vi "Global_Device_IDs.vi"() -> ()   [LabVIEW 2017]
uses:
  TypeDef/CLUSTER_Claw_Setup.ctl
  TypeDef/CLUSTER_PWM Motor Setup.ctl
  TypeDef/CLUSTER_Solonoid_Setup.ctl
  <vilib>/Rock Robotics/WPI/Solenoid/WPI_SolenoidChannel.ctl
  <vilib>/Rock Robotics/SystemInterfaces/DIO/FPGA_DIOChannel.ctl
  TypeDef/CLUSTER_Arm_Device_IDs.ctl
  TypeDef/CLUSTER_Talon_Setup.ctl
  _SHARE ALL/RoboRio Share All/SRX Share All/TypeDefs SRX/Cluster_SRX_OPEN Data.ctl
  _SHARE ALL/RoboRio Share All/SRX Share All/TypeDefs SRX/Cluster_SRX_Current Config.ctl
  _SHARE ALL/RoboRio Share All/SRX Share All/TypeDefs SRX/Cluster_SRX_Sensor Config.ctl
  System Drivers/Phoenix-LabVIEW/Motor Controller/Controls/CTRE_Phoenix_MotorControl_FeedbackDevice.ctl
  _SHARE ALL/RoboRio Share All/SRX Share All/TypeDefs SRX/Cluster_SRX_Config Hard Limits.ctl
  System Drivers/Phoenix-LabVIEW/Motor Controller/Controls/CTRE_Phoenix_MotorControl_LimitSwitchNormal.ctl
  _SHARE ALL/RoboRio Share All/SRX Share All/TypeDefs SRX/Cluster_SRX_Motion Magic Config Data.ctl
  _SHARE ALL/RoboRio Share All/SRX Share All/TypeDefs SRX/Cluster_SRX_PIDF.ctl
  _SHARE ALL/RoboRio Share All/SRX Share All/TypeDefs SRX/Cluster_SRX_Config Soft Limits.ctl
  _SHARE ALL/RoboRio Share All/SRX Share All/TypeDefs SRX/Cluster_SRX_Config Voltage Output.ctl
  System Drivers/Phoenix-LabVIEW/Motor Controller/Controls/CTRE_Phoenix_MotorControl_NeutralMode.ctl
  _SHARE ALL/RoboRio Share All/SRX Share All/TypeDefs SRX/Cluster_SRX_Forward and Reverse.ctl
  TypeDef/CLUSTER_Drive_Setup.ctl
panel:
  in  "Drive Setup":T1={"Left Master"={"Open Data"={"SRX ID"=0, "Invert Output"=FALSE}, "Current Config Data"={"Enable Current Limit?"=FALSE, "Peak Current (Amps)"=0, "Peak Current Maximum Duration (ms)"=0, "Continuous Current Limit (Amps)"=0}, "Sensor Config"={"Feedback Device"=1, "PhaseSensor"=FALSE}, "Hard Limits"={"Fwd Enable"=FALSE, "Rev Enable"=FALSE, "Fwd NO-NC"=enum."Normally Open", "Rev NO-NC"=enum."Normally Open"}, "Motion Magic Config Data"={"Cruise Velocity"=0, "Acceleration"=0}, "PIDF"={"P"=0.0, "I"=0.0, "D"=0.0, "F"=0.0, "I Zone"=0.0}, "Maximum Integral Accumulator Value"=0.0, "AllowableClosedLoop"=0, "Limits"={"Max"=0, "Min"=0, "Max Enable"=FALSE, "Min Enable"=FALSE}, "Output Config"={"Invert?"=FALSE, "Neutral Mode"=enum."EEPROMSetting", "Deadband (-1to1)"=0.0, "Ramp Time Off to Full (S)"=0.0, "Peak  (-1to1)"={"Forward"=1.0, "Reverse"=-1.0}, "Nominal  (-1to1)"={"Forward"=0.0, "Reverse"=0.0}}}, "Right Master"={"Open Data"={"SRX ID"=0, "Invert Output"=FALSE}, "Current Config Data"={"Enable Current Limit?"=FALSE, "Peak Current (Amps)"=0, "Peak Current Maximum Duration (ms)"=0, "Continuous Current Limit (Amps)"=0}, "Sensor Config"={"Feedback Device"=1, "PhaseSensor"=FALSE}, "Hard Limits"={"Fwd Enable"=FALSE, "Rev Enable"=FALSE, "Fwd NO-NC"=enum."Normally Open", "Rev NO-NC"=enum."Normally Open"}, "Motion Magic Config Data"={"Cruise Velocity"=0, "Acceleration"=0}, "PIDF"={"P"=0.0, "I"=0.0, "D"=0.0, "F"=0.0, "I Zone"=0.0}, "Maximum Integral Accumulator Value"=0.0, "AllowableClosedLoop"=0, "Limits"={"Max"=0, "Min"=0, "Max Enable"=FALSE, "Min Enable"=FALSE}, "Output Config"={"Invert?"=FALSE, "Neutral Mode"=enum."EEPROMSetting", "Deadband (-1to1)"=0.0, "Ramp Time Off to Full (S)"=0.0, "Peak  (-1to1)"={"Forward"=1.0, "Reverse"=-1.0}, "Nominal  (-1to1)"={"Forward"=0.0, "Reverse"=0.0}}}, "Left Slave"={"Open Data"={"SRX ID"=0, "Invert Output"=FALSE}, "Current Config Data"={"Enable Current Limit?"=FALSE, "Peak Current (Amps)"=0, "Peak Current Maximum Duration (ms)"=0, "Continuous Current Limit (Amps)"=0}, "Sensor Config"={"Feedback Device"=1, "PhaseSensor"=FALSE}, "Hard Limits"={"Fwd Enable"=FALSE, "Rev Enable"=FALSE, "Fwd NO-NC"=enum."Normally Open", "Rev NO-NC"=enum."Normally Open"}, "Motion Magic Config Data"={"Cruise Velocity"=0, "Acceleration"=0}, "PIDF"={"P"=0.0, "I"=0.0, "D"=0.0, "F"=0.0, "I Zone"=0.0}, "Maximum Integral Accumulator Value"=0.0, "AllowableClosedLoop"=0, "Limits"={"Max"=0, "Min"=0, "Max Enable"=FALSE, "Min Enable"=FALSE}, "Output Config"={"Invert?"=FALSE, "Neutral Mode"=enum."EEPROMSetting", "Deadband (-1to1)"=0.0, "Ramp Time Off to Full (S)"=0.0, "Peak  (-1to1)"={"Forward"=1.0, "Reverse"=-1.0}, "Nominal  (-1to1)"={"Forward"=0.0, "Reverse"=0.0}}}, "Right Slave"={"Open Data"={"SRX ID"=0, "Invert Output"=FALSE}, "Current Config Data"={"Enable Current Limit?"=FALSE, "Peak Current (Amps)"=0, "Peak Current Maximum Duration (ms)"=0, "Continuous Current Limit (Amps)"=0}, "Sensor Config"={"Feedback Device"=1, "PhaseSensor"=FALSE}, "Hard Limits"={"Fwd Enable"=FALSE, "Rev Enable"=FALSE, "Fwd NO-NC"=enum."Normally Open", "Rev NO-NC"=enum."Normally Open"}, "Motion Magic Config Data"={"Cruise Velocity"=0, "Acceleration"=0}, "PIDF"={"P"=0.0, "I"=0.0, "D"=0.0, "F"=0.0, "I Zone"=0.0}, "Maximum Integral Accumulator Value"=0.0, "AllowableClosedLoop"=0, "Limits"={"Max"=0, "Min"=0, "Max Enable"=FALSE, "Min Enable"=FALSE}, "Output Config"={"Invert?"=FALSE, "Neutral Mode"=enum."EEPROMSetting", "Deadband (-1to1)"=0.0, "Ramp Time Off to Full (S)"=0.0, "Peak  (-1to1)"={"Forward"=1.0, "Reverse"=-1.0}, "Nominal  (-1to1)"={"Forward"=0.0, "Reverse"=0.0}}}, "Left Slave Top"={"Open Data"={"SRX ID"=0, "Invert Output"=FALSE}, "Current Config Data"={"Enable Current Limit?"=FALSE, "Peak Current (Amps)"=0, "Peak Current Maximum Duration (ms)"=0, "Continuous Current Limit (Amps)"=0}, "Sensor Config"={"Feedback Device"=1, "PhaseSensor"=FALSE}, "Hard Limits"={"Fwd Enable"=FALSE, "Rev Enable"=FALSE, "Fwd NO-NC"=enum."Normally Open", "Rev NO-NC"=enum."Normally Open"}, "Motion Magic Config Data"={"Cruise Velocity"=0, "Acceleration"=0}, "PIDF"={"P"=0.0, "I"=0.0, "D"=0.0, "F"=0.0, "I Zone"=0.0}, "Maximum Integral Accumulator Value"=0.0, "AllowableClosedLoop"=0, "Limits"={"Max"=0, "Min"=0, "Max Enable"=FALSE, "Min Enable"=FALSE}, "Output Config"={"Invert?"=FALSE, "Neutral Mode"=enum."EEPROMSetting", "Deadband (-1to1)"=0.0, "Ramp Time Off to Full (S)"=0.0, "Peak  (-1to1)"={"Forward"=1.0, "Reverse"=-1.0}, "Nominal  (-1to1)"={"Forward"=0.0, "Reverse"=0.0}}}, "Right Slave Top"={"Open Data"={"SRX ID"=0, "Invert Output"=FALSE}, "Current Config Data"={"Enable Current Limit?"=FALSE, "Peak Current (Amps)"=0, "Peak Current Maximum Duration (ms)"=0, "Continuous Current Limit (Amps)"=0}, "Sensor Config"={"Feedback Device"=1, "PhaseSensor"=FALSE}, "Hard Limits"={"Fwd Enable"=FALSE, "Rev Enable"=FALSE, "Fwd NO-NC"=enum."Normally Open", "Rev NO-NC"=enum."Normally Open"}, "Motion Magic Config Data"={"Cruise Velocity"=0, "Acceleration"=0}, "PIDF"={"P"=0.0, "I"=0.0, "D"=0.0, "F"=0.0, "I Zone"=0.0}, "Maximum Integral Accumulator Value"=0.0, "AllowableClosedLoop"=0, "Limits"={"Max"=0, "Min"=0, "Max Enable"=FALSE, "Min Enable"=FALSE}, "Output Config"={"Invert?"=FALSE, "Neutral Mode"=enum."EEPROMSetting", "Deadband (-1to1)"=0.0, "Ramp Time Off to Full (S)"=0.0, "Peak  (-1to1)"={"Forward"=1.0, "Reverse"=-1.0}, "Nominal  (-1to1)"={"Forward"=0.0, "Reverse"=0.0}}}} {"Right Slave Top"."Sensor Config"."Feedback Device" items=["None"=-1, "QuadEncoder"=0, "Analog"=2, "Tachometer"=4, "Pulse Width Encoded Position"=8, "Sensor Sum (S0 + S1)"=9, "Sensor Difference (D0 - D1)"=10, "Remote Source 0"=11, "Remote Source 1"=12, "Software Emulated"=15]; "Left Slave Top"."Sensor Config"."Feedback Device" items=["None"=-1, "QuadEncoder"=0, "Analog"=2, "Tachometer"=4, "Pulse Width Encoded Position"=8, "Sensor Sum (S0 + S1)"=9, "Sensor Difference (D0 - D1)"=10, "Remote Source 0"=11, "Remote Source 1"=12, "Software Emulated"=15]; "Left Master"."Sensor Config"."Feedback Device" items=["None"=-1, "QuadEncoder"=0, "Analog"=2, "Tachometer"=4, "Pulse Width Encoded Position"=8, "Sensor Sum (S0 + S1)"=9, "Sensor Difference (D0 - D1)"=10, "Remote Source 0"=11, "Remote Source 1"=12, "Software Emulated"=15]; "Right Master"."Sensor Config"."Feedback Device" items=["None"=-1, "QuadEncoder"=0, "Analog"=2, "Tachometer"=4, "Pulse Width Encoded Position"=8, "Sensor Sum (S0 + S1)"=9, "Sensor Difference (D0 - D1)"=10, "Remote Source 0"=11, "Remote Source 1"=12, "Software Emulated"=15]; "Left Slave"."Sensor Config"."Feedback Device" items=["None"=-1, "QuadEncoder"=0, "Analog"=2, "Tachometer"=4, "Pulse Width Encoded Position"=8, "Sensor Sum (S0 + S1)"=9, "Sensor Difference (D0 - D1)"=10, "Remote Source 0"=11, "Remote Source 1"=12, "Software Emulated"=15]; "Right Slave"."Sensor Config"."Feedback Device" items=["None"=-1, "QuadEncoder"=0, "Analog"=2, "Tachometer"=4, "Pulse Width Encoded Position"=8, "Sensor Sum (S0 + S1)"=9, "Sensor Difference (D0 - D1)"=10, "Remote Source 0"=11, "Remote Source 1"=12, "Software Emulated"=15]}
  out "Claw Rotation Setup":T2={"Open Data"={"SRX ID"=0, "Invert Output"=FALSE}, "Current Config Data"={"Enable Current Limit?"=FALSE, "Peak Current (Amps)"=0, "Peak Current Maximum Duration (ms)"=0, "Continuous Current Limit (Amps)"=0}, "Sensor Config"={"Feedback Device"=0, "PhaseSensor"=FALSE}, "Hard Limits"={"Fwd Enable"=FALSE, "Rev Enable"=FALSE, "Fwd NO-NC"=enum."Normally Open", "Rev NO-NC"=enum."Normally Open"}, "Motion Magic Config Data"={"Cruise Velocity"=0, "Acceleration"=0}, "PIDF"={"P"=0.0, "I"=0.0, "D"=0.0, "F"=0.0, "I Zone"=0.0}, "Maximum Integral Accumulator Value"=0.0, "AllowableClosedLoop"=0, "Limits"={"Max"=0, "Min"=0, "Max Enable"=FALSE, "Min Enable"=FALSE}, "Output Config"={"Invert?"=FALSE, "Neutral Mode"=enum."Override to Coast", "Deadband (-1to1)"=0.0, "Ramp Time Off to Full (S)"=0.0, "Peak  (-1to1)"={"Forward"=1.0, "Reverse"=-1.0}, "Nominal  (-1to1)"={"Forward"=0.0, "Reverse"=0.0}}} {"Sensor Config"."Feedback Device" items=["None"=-1, "QuadEncoder"=0, "Analog"=2, "Tachometer"=4, "Pulse Width Encoded Position"=8, "Sensor Sum (S0 + S1)"=9, "Sensor Difference (D0 - D1)"=10, "Remote Source 0"=11, "Remote Source 1"=12, "Software Emulated"=15]}
  in  "Lift Setup":T15={"Master"={"Open Data"={"SRX ID"=0, "Invert Output"=FALSE}, "Current Config Data"={"Enable Current Limit?"=FALSE, "Peak Current (Amps)"=0, "Peak Current Maximum Duration (ms)"=2, "Continuous Current Limit (Amps)"=0}, "Sensor Config"={"Feedback Device"=0, "PhaseSensor"=FALSE}, "Hard Limits"={"Fwd Enable"=FALSE, "Rev Enable"=FALSE, "Fwd NO-NC"=enum."Normally Open", "Rev NO-NC"=enum."Normally Open"}, "Motion Magic Config Data"={"Cruise Velocity"=0, "Acceleration"=0}, "PIDF"={"P"=0.0, "I"=0.0, "D"=0.0, "F"=0.0, "I Zone"=0.0}, "Maximum Integral Accumulator Value"=0.0, "AllowableClosedLoop"=0, "Limits"={"Max"=0, "Min"=0, "Max Enable"=FALSE, "Min Enable"=FALSE}, "Output Config"={"Invert?"=FALSE, "Neutral Mode"=enum."Override to Coast", "Deadband (-1to1)"=0.0, "Ramp Time Off to Full (S)"=0.0, "Peak  (-1to1)"={"Forward"=1.0, "Reverse"=-1.0}, "Nominal  (-1to1)"={"Forward"=0.0, "Reverse"=0.0}}}, "Slave"={"Open Data"={"SRX ID"=0, "Invert Output"=FALSE}, "Current Config Data"={"Enable Current Limit?"=FALSE, "Peak Current (Amps)"=0, "Peak Current Maximum Duration (ms)"=-1, "Continuous Current Limit (Amps)"=0}, "Sensor Config"={"Feedback Device"=0, "PhaseSensor"=FALSE}, "Hard Limits"={"Fwd Enable"=FALSE, "Rev Enable"=FALSE, "Fwd NO-NC"=enum."Normally Open", "Rev NO-NC"=enum."Normally Open"}, "Motion Magic Config Data"={"Cruise Velocity"=0, "Acceleration"=0}, "PIDF"={"P"=0.0, "I"=0.0, "D"=0.0, "F"=0.0, "I Zone"=0.0}, "Maximum Integral Accumulator Value"=0.0, "AllowableClosedLoop"=0, "Limits"={"Max"=0, "Min"=0, "Max Enable"=FALSE, "Min Enable"=FALSE}, "Output Config"={"Invert?"=FALSE, "Neutral Mode"=enum."Override to Coast", "Deadband (-1to1)"=0.0, "Ramp Time Off to Full (S)"=0.0, "Peak  (-1to1)"={"Forward"=1.0, "Reverse"=-1.0}, "Nominal  (-1to1)"={"Forward"=0.0, "Reverse"=0.0}}}} {"Slave"."Sensor Config"."Feedback Device" items=["None"=-1, "QuadEncoder"=0, "Analog"=2, "Tachometer"=4, "Pulse Width Encoded Position"=8, "Sensor Sum (S0 + S1)"=9, "Sensor Difference (D0 - D1)"=10, "Remote Source 0"=11, "Remote Source 1"=12, "Software Emulated"=15]; "Master"."Sensor Config"."Feedback Device" items=["None"=-1, "QuadEncoder"=0, "Analog"=2, "Tachometer"=4, "Pulse Width Encoded Position"=8, "Sensor Sum (S0 + S1)"=9, "Sensor Difference (D0 - D1)"=10, "Remote Source 0"=11, "Remote Source 1"=12, "Software Emulated"=15]}
  in  "Arm Setup":T15={"Master"={"Open Data"={"SRX ID"=0, "Invert Output"=FALSE}, "Current Config Data"={"Enable Current Limit?"=FALSE, "Peak Current (Amps)"=0, "Peak Current Maximum Duration (ms)"=2, "Continuous Current Limit (Amps)"=0}, "Sensor Config"={"Feedback Device"=0, "PhaseSensor"=FALSE}, "Hard Limits"={"Fwd Enable"=FALSE, "Rev Enable"=FALSE, "Fwd NO-NC"=enum."Normally Open", "Rev NO-NC"=enum."Normally Open"}, "Motion Magic Config Data"={"Cruise Velocity"=0, "Acceleration"=0}, "PIDF"={"P"=0.0, "I"=0.0, "D"=0.0, "F"=0.0, "I Zone"=0.0}, "Maximum Integral Accumulator Value"=0.0, "AllowableClosedLoop"=0, "Limits"={"Max"=0, "Min"=0, "Max Enable"=FALSE, "Min Enable"=FALSE}, "Output Config"={"Invert?"=FALSE, "Neutral Mode"=enum."Override to Coast", "Deadband (-1to1)"=0.0, "Ramp Time Off to Full (S)"=0.0, "Peak  (-1to1)"={"Forward"=1.0, "Reverse"=-1.0}, "Nominal  (-1to1)"={"Forward"=0.0, "Reverse"=0.0}}}, "Slave"={"Open Data"={"SRX ID"=0, "Invert Output"=FALSE}, "Current Config Data"={"Enable Current Limit?"=FALSE, "Peak Current (Amps)"=0, "Peak Current Maximum Duration (ms)"=-1, "Continuous Current Limit (Amps)"=0}, "Sensor Config"={"Feedback Device"=0, "PhaseSensor"=FALSE}, "Hard Limits"={"Fwd Enable"=FALSE, "Rev Enable"=FALSE, "Fwd NO-NC"=enum."Normally Open", "Rev NO-NC"=enum."Normally Open"}, "Motion Magic Config Data"={"Cruise Velocity"=0, "Acceleration"=0}, "PIDF"={"P"=0.0, "I"=0.0, "D"=0.0, "F"=0.0, "I Zone"=0.0}, "Maximum Integral Accumulator Value"=0.0, "AllowableClosedLoop"=0, "Limits"={"Max"=0, "Min"=0, "Max Enable"=FALSE, "Min Enable"=FALSE}, "Output Config"={"Invert?"=FALSE, "Neutral Mode"=enum."Override to Coast", "Deadband (-1to1)"=0.0, "Ramp Time Off to Full (S)"=0.0, "Peak  (-1to1)"={"Forward"=1.0, "Reverse"=-1.0}, "Nominal  (-1to1)"={"Forward"=0.0, "Reverse"=0.0}}}} {"Slave"."Sensor Config"."Feedback Device" items=["None"=-1, "QuadEncoder"=0, "Analog"=2, "Tachometer"=4, "Pulse Width Encoded Position"=8, "Sensor Sum (S0 + S1)"=9, "Sensor Difference (D0 - D1)"=10, "Remote Source 0"=11, "Remote Source 1"=12, "Software Emulated"=15]; "Master"."Sensor Config"."Feedback Device" items=["None"=-1, "QuadEncoder"=0, "Analog"=2, "Tachometer"=4, "Pulse Width Encoded Position"=8, "Sensor Sum (S0 + S1)"=9, "Sensor Difference (D0 - D1)"=10, "Remote Source 0"=11, "Remote Source 1"=12, "Software Emulated"=15]}
  in  "Claw Setup":T16={"Left Motor Setup"={"Motor ID"=20, "Invert Motor"=FALSE}, "Right Motor Setup"={"Motor ID"=20, "Invert Motor"=FALSE}, "Left Motor PDP"=0, "Right Motor PDP"=0, "Solonoid Setup"={"Pneumatics Control Module (0)"=0, "Solenoid Channel"=enum."Solenoid 0"}, "Limit Switch DIO"=enum."DIO 0"}
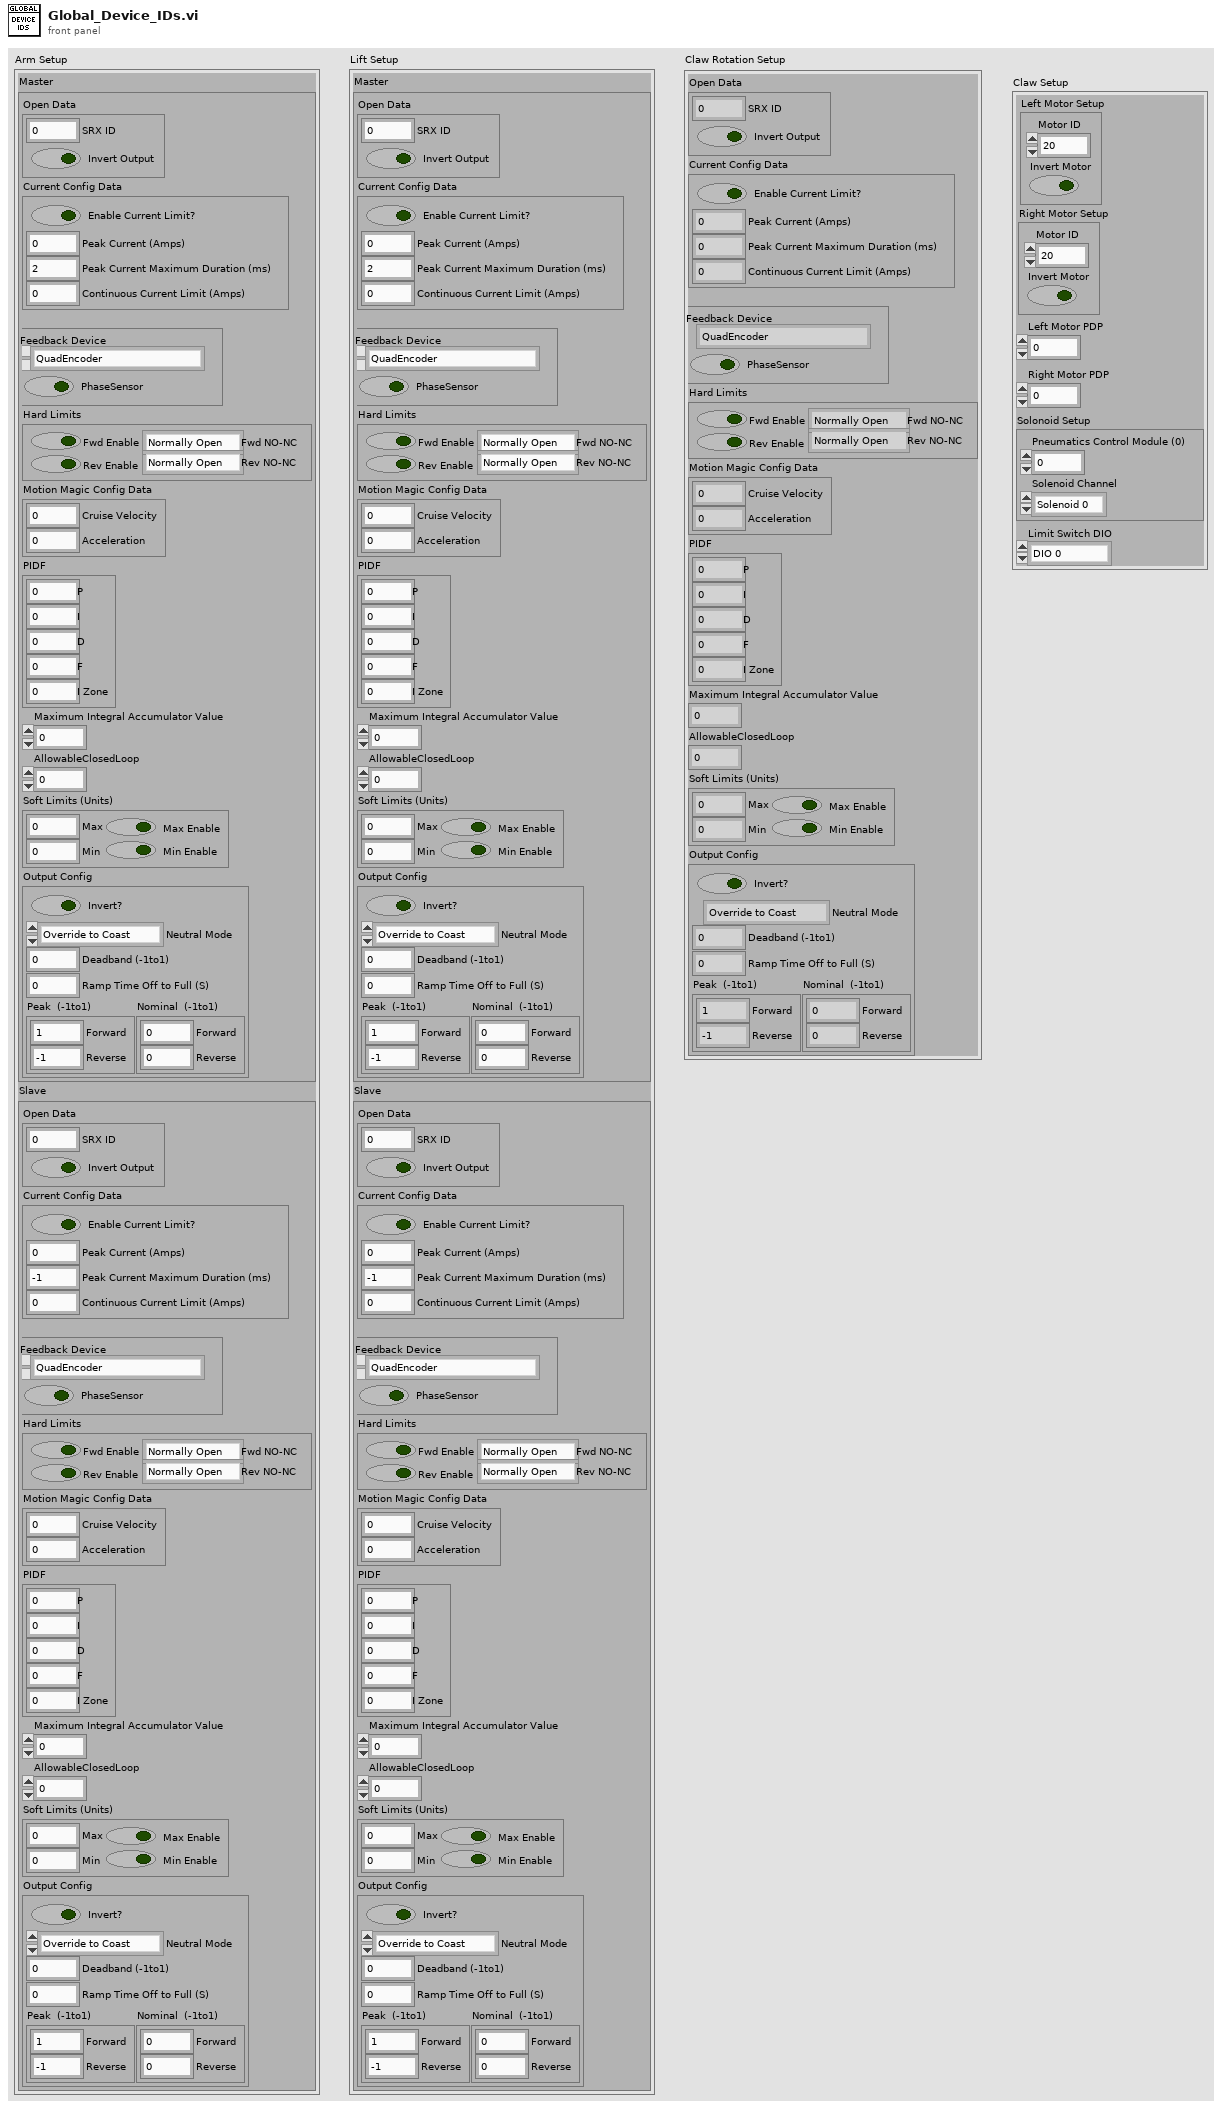
[diagram p1: front panel]
types:
  T1 = typedef "CLUSTER_Drive_Setup.ctl" = cluster{"Left Master":T2, "Right Master":T2, "Left Slave":T2, "Right Slave":T2, "Left Slave Top":T2, "Right Slave Top":T2}
  T2 = typedef "CLUSTER_Talon_Setup.ctl" = cluster{"Open Data":T3, "Current Config Data":T4, "Sensor Config":T5, "Hard Limits":T7, "Motion Magic Config Data":T9, "PIDF":T10, "Maximum Integral Accumulator Value":dbl, "AllowableClosedLoop":i32, "Limits":T11, "Output Config":T12}
  T3 = typedef "Cluster_SRX_OPEN Data.ctl" = cluster{"SRX ID":u8, "Invert Output":bool}
  T4 = typedef "Cluster_SRX_Current Config.ctl" = cluster{"Enable Current Limit?":bool, "Peak Current (Amps)":i32, "Peak Current Maximum Duration (ms)":i32, "Continuous Current Limit (Amps)":i32}
  T5 = typedef "Cluster_SRX_Sensor Config.ctl" = cluster{"Feedback Device":T6, "PhaseSensor":bool}
  T6 = typedef "CTRE_Phoenix_MotorControl_FeedbackDevice.ctl" = i8
  T7 = typedef "Cluster_SRX_Config Hard Limits.ctl" = cluster{"Fwd Enable":bool, "Rev Enable":bool, "Fwd NO-NC":T8, "Rev NO-NC":T8}
  T8 = typedef "CTRE_Phoenix_MotorControl_LimitSwitchNormal.ctl" = enum16{"Normally Open", "Normally Closed", "Disabled"}
  T9 = typedef "Cluster_SRX_Motion Magic Config Data.ctl" = cluster{"Cruise Velocity":i32, "Acceleration":i32}
  T10 = typedef "Cluster_SRX_PIDF.ctl" = cluster{"P":dbl, "I":dbl, "D":dbl, "F":dbl, "I Zone":dbl}
  T11 = typedef "Cluster_SRX_Config Soft Limits.ctl" = cluster{"Max":i32, "Min":i32, "Max Enable":bool, "Min Enable":bool}
  T12 = typedef "Cluster_SRX_Config Voltage Output.ctl" = cluster{"Invert?":bool, "Neutral Mode":T13, "Deadband (-1to1)":dbl, "Ramp Time Off to Full (S)":dbl, "Peak  (-1to1)":T14, "Nominal  (-1to1)":T14}
  T13 = typedef "CTRE_Phoenix_MotorControl_NeutralMode.ctl" = enum8{"EEPROMSetting", "Override to Coast", "Override to Brake"}
  T14 = typedef "Cluster_SRX_Forward and Reverse.ctl" = cluster{"Forward":dbl, "Reverse":dbl}
  T15 = typedef "CLUSTER_Arm_Device_IDs.ctl" = cluster{"Master":T2, "Slave":T2}
  T16 = typedef "CLUSTER_Claw_Setup.ctl" = cluster{"Left Motor Setup":T17, "Right Motor Setup":T17, "Left Motor PDP":i32, "Right Motor PDP":i32, "Solonoid Setup":T18, "Limit Switch DIO":T20}
  T17 = typedef "CLUSTER_PWM Motor Setup.ctl" = cluster{"Motor ID":u8, "Invert Motor":bool}
  T18 = typedef "CLUSTER_Solonoid_Setup.ctl" = cluster{"Pneumatics Control Module (0)":u8, "Solenoid Channel":T19}
  T19 = typedef "WPI_SolenoidChannel.ctl" = enum8{"Solenoid 0", "Solenoid 1", "Solenoid 2", "Solenoid 3", "Solenoid 4", "Solenoid 5", "Solenoid 6", "Solenoid 7", "Invalid"}
  T20 = typedef "FPGA_DIOChannel.ctl" = enum8{"DIO 0", "DIO 1", "DIO 2", "DIO 3", "DIO 4", "DIO 5", "DIO 6", "DIO 7", "DIO 8", "DIO 9", "DIO MXP 0", "DIO MXP 1", "DIO MXP 2", "DIO MXP 3", "DIO MXP 4", "DIO MXP 5", "DIO MXP 6", "DIO MXP 7", "DIO MXP 8", "DIO MXP 9", "DIO MXP 10", "DIO MXP 11", "DIO MXP 12", "DIO MXP 13", "DIO MXP 14", "DIO MXP 15", "SPI Port CS1", "SPI Port CS2", "SPI Port CS3", "SPI Port MISO", "SPI Port MOSI", "Invalid"}
diagram:
